vi "ACT_Loop.vi"() -> ()   [LabVIEW 2023, in "TShirtWork-SwerveDrive_ACT_ts.lvlib"]
uses:
  TShirtWork-SwerveDrive_ACT_ts.lvlib
  RoboRIO Utilities/Global_STOP.vi
  ENUM_ACT_Action.ctl
  ENUM_ACT_State.ctl
  Global_CMD_ACT_Data In.vi
  Global_ACT_Data Out.vi
  Cluster_CMD_ACT_Data.ctl
  <vilib>/Rock Robotics/WPI/MotorControl/WPI_MotorControlType.ctl
  <vilib>/Rock Robotics/SystemInterfaces/DIO/FPGA_DIOPWMChannel.ctl
  <vilib>/Rock Robotics/WPI/PWM/WPI_PWMDeadband.ctl
  <vilib>/Rock Robotics/SystemInterfaces/DIO/FPGA_DIOChannel.ctl
  <vilib>/Rock Robotics/WPI/MotorControl/WPI_MotorControlDeviceRef.ctl
  Shared Code/TypeDefs/ENUM_Module Position.ctl
  <vilib>/Rock Robotics/WPI/ThirdParty/REV Robotics/REVLib/Typedef/Spark MAX Control Type.ctl
  Type Defs/ENUM_Steer Mode Select.ctl
  Shared Code/TypeDefs/Cluster_CMD_Direction Data.ctl
  Shared Code/TypeDefs/Level_Velocity plus-minus 1.ctl
  Shared Code/TypeDefs/Dial_Compase heading unit circle CCW positive.ctl
  Shared Code/TypeDefs/Cluster_Module Velocity-Direction-Rotations.ctl
  Shared Code/TypeDefs/Cluster_Swerve 4 Steer and Velocity.ctl
  Shared Code/TypeDefs/Cluster_X-Y.ctl
  Type Defs/Cluster_Avoid Zone.ctl
  PigeonIMU/Global_SEN_Data Out.vi
  PigeonIMU/PigeonIMU_SEN_ts.lvlib
  Shared Code/TypeDefs/Cluster_Config_SwerveParam Drive.ctl
  Type Defs/Cluster_Length and Width.ctl
  Shared Code/TypeDefs/Cluster_Config_SwerveParam Steer.ctl
  Shared Code/TypeDefs/Cluster_Config_Swerve Drive Parameters.ctl
  Shared Code/TypeDefs/ENUM_CMD_Mode Select.ctl
  <vilib>/Rock Robotics/WPI/ThirdParty/Phoenix-LabVIEW/Motor Controller/Get/CTRE_Phoenix_MotorController_GetSelectedSensorData.vi
  Shared Code/TypeDefs/ENUM_Min Max Values.ctl
  Type Defs/Cluster_Zero Steer Positions.ctl
  Shared Code/TypeDefs/Dial_Actual Direction.ctl
  Shared Code/TypeDefs/Cluster_Module Actual Settings.ctl
  Shared Code/TypeDefs/Cluster_Swerve Actual Settings.ctl
panel:
  out "Yaw":T1 scale format="%.3f"
  out "Swerve SET Actual":T2 {"Back Right"."Direction" scale format="%.3f"; "Back Right"."Velocity" format="%.2f"; "Back Left"."Direction" scale format="%.3f"; "Back Left"."Velocity" format="%.2f"; "Front Left"."Direction" scale format="%.3f"; "Front Left"."Velocity" format="%.2f"; "Front Right"."Direction" scale format="%.3f"; "Front Right"."Velocity" format="%.2f"}
  out "calc time":dbl
  in  "Zero Steer Positions":T5 {"RB"."Max" format="%.3g"; "RB"."Min" format="%.3g"; "LB"."Max" format="%.3g"; "LB"."Min" format="%.3g"; "LF"."Max" format="%.3g"; "LF"."Min" format="%.3g"; "RF"."Max" format="%.3g"; "RF"."Min" format="%.3g"}
  out "Swerve Set":T7 {"Back Right"."Angle" scale format="%.3f"; "Back Right"."Velocity" scale=-1.0..1.0 scale format="%.1f"; "Back Left"."Angle" scale format="%.3f"; "Back Left"."Velocity" scale=-1.0..1.0 scale format="%.1f"; "Front Left"."Angle" scale format="%.3f"; "Front Left"."Velocity" scale=-1.0..1.0 scale format="%.1f"; "Front Right"."Angle" scale format="%.3f"; "Front Right"."Velocity" scale=-1.0..1.0 scale format="%.1f"}
  out "Max Velocity(RPM)":dbl=200.0
  out "Steer Mode":T10
  out "Max Velocity FPS":dbl=2.0
  out "Steer Position Values":dbl[](array[numeric])
  out "Drive Control Mode":T11
  in  "Stream":bool=TRUE
  out "Input CMD":T12 {"Auto Angle" scale format="%.3f"; "Direction"."Rotate(Yaw) CCW 1 CW -1" scale=1.0..-1.0; "Direction"."Traverse"."Angle" scale format="%.3f"; "Direction"."Traverse"."Velocity" scale=-1.0..1.0 scale format="%.1f"}
  out "Cycle Time (S)":dbl format="%.3g"
  # "\"Front\" of Robot"
  # "X"
  # "+CCW"
  # "Y"
  # "(0,0)"
  # "\"Front\" of Robot"
  # "Right Hand Rule"
  # "X"
  # "+CCW"
  # "Y"
  # "(0,0)"
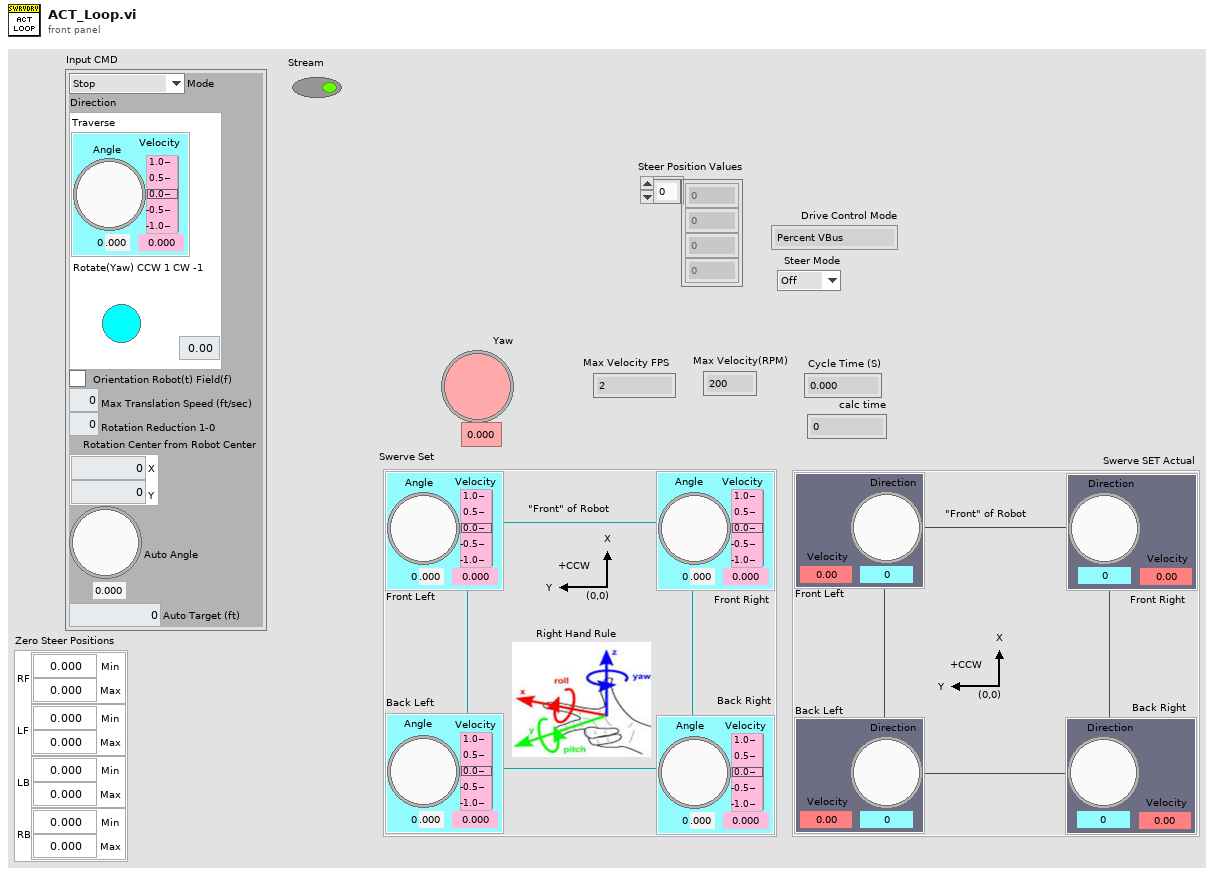
[diagram p1: front panel]
types:
  T1 = typedef "Dial_Compase heading unit circle CCW positive.ctl" = dbl
  T2 = typedef "Cluster_Swerve Actual Settings.ctl" = cluster{"Front Right":T3, "Front Left":T3, "Back Left":T3, "Back Right":T3}
  T3 = typedef "Cluster_Module Actual Settings.ctl" = cluster{"Velocity":dbl, "Direction":T4, "Encoder":dbl}
  T4 = typedef "Dial_Actual Direction.ctl" = dbl
  T5 = typedef "Cluster_Zero Steer Positions.ctl" = cluster{"RF":T6, "LF":T6, "LB":T6, "RB":T6}
  T6 = typedef "ENUM_Min Max Values.ctl" = cluster{"Min":dbl, "Max":dbl}
  T7 = typedef "Cluster_Swerve 4 Steer and Velocity.ctl" = cluster{"Front Right":T8, "Front Left":T8, "Back Left":T8, "Back Right":T8}
  T8 = typedef "Cluster_Module Velocity-Direction-Rotations.ctl" = cluster{"Velocity":T9, "Angle":T1, "Rotations Count":dbl}
  T9 = typedef "Level_Velocity plus-minus 1.ctl" = dbl
  T10 = typedef "ENUM_Steer Mode Select.ctl" = enum16{"Off", "Hold", "Steer"}
  T11 = typedef "Spark MAX Control Type.ctl" = enum16{"Percent VBus", "Voltage", "Velocity", "Position", "Smart Motion", "Current", "Smart Velocity"}
  T12 = typedef "TShirtWork-SwerveDrive_ACT_ts.lvlib/Cluster_CMD_ACT_Data.ctl" = cluster{"Mode":T13, "Direction":T14, "Orientation Robot(t) Field(f)":bool, "Max Translation Speed (ft/sec)":dbl, "Rotation Reduction 1-0":dbl, "Rotation Center from Robot Center":T15, "Auto Angle":T1, "Auto Target (ft)":dbl}
  T13 = typedef "ENUM_CMD_Mode Select.ctl" = enum16{"Stop", "Move", "Turret Manual"}
  T14 = typedef "Cluster_CMD_Direction Data.ctl" = cluster{"Traverse":T8, "Rotate(Yaw) CCW 1 CW -1":dbl}
  T15 = typedef "Cluster_X-Y.ctl" = cluster{"X":dbl, "Y":dbl}
  T16 = typedef "Cluster_Config_Swerve Drive Parameters.ctl" = cluster{"SwerveParam Ver":u64, "Frame":T17, "Steer":T18, "Drive":T19}
  T17 = typedef "Cluster_Length and Width.ctl" = cluster{"Length":dbl, "Width":dbl}
  T18 = typedef "Cluster_Config_SwerveParam Steer.ctl" = cluster{"CPR":dbl}
  T19 = typedef "Cluster_Config_SwerveParam Drive.ctl" = cluster{"CPR":dbl, "RevMotor/Wheel":dbl, "Wheel Diameter (in)":dbl}
  T20 = typedef "Cluster_Avoid Zone.ctl" = cluster{"pos 1":dbl, "pos 2":dbl}
  T21 = typedef "ENUM_Module Position.ctl" = enum16{"Left-Front", "Right-Front", "Left-Back", "Right-Back"}
  T22 = typedef "WPI_MotorControlDeviceRef.ctl" = cluster{"DeviceStatus":errorcluster, "Type":T23, "PWM":cluster{"PWM Channel":T24, "DeadBand":T25}, "CAN":cluster{"Device Number":u8, "SetOutput VI Ref":variant, "GetOutput VI Ref":variant, "Enable VI Ref":variant, "Disable VI Ref":variant, "Data":variant}, "Invert":bool, "DIO PWM":cluster{"PWM \"Enable\" Channel":T24, "DIOChannel":T26, "PWM Rate":dbl}}
  T23 = typedef "WPI_MotorControlType.ctl" = enum16{"PWM", "CAN", "DIO PWM"}
  T24 = typedef "FPGA_DIOPWMChannel.ctl" = enum8{"PWM 0", "PWM 1", "PWM 2", "PWM 3", "PWM 4", "PWM 5", "PWM 6", "PWM 7", "PWM 8", "PWM 9", "PWM MXP 0", "PWM MXP 1", "PWM MXP 2", "PWM MXP 3", "PWM MXP 4", "PWM MXP 5", "PWM MXP 6", "PWM MXP 7", "PWM MXP 8", "PWM MXP 9", "Invalid"}
  T25 = typedef "WPI_PWMDeadband.ctl" = cluster{"Name":string, "maxPositivePwm":i32, "minPositivePwm":i32, "centerPwm":i32, "maxNegativePwm":i32, "minNegativePwm":i32, "angularRange":u16}
  T26 = typedef "FPGA_DIOChannel.ctl" = enum8{"DIO 0", "DIO 1", "DIO 2", "DIO 3", "DIO 4", "DIO 5", "DIO 6", "DIO 7", "DIO 8", "DIO 9", "DIO MXP 0", "DIO MXP 1", "DIO MXP 2", "DIO MXP 3", "DIO MXP 4", "DIO MXP 5", "DIO MXP 6", "DIO MXP 7", "DIO MXP 8", "DIO MXP 9", "DIO MXP 10", "DIO MXP 11", "DIO MXP 12", "DIO MXP 13", "DIO MXP 14", "DIO MXP 15", "SPI Port CS1", "SPI Port CS2", "SPI Port CS3", "SPI Port MISO", "SPI Port MOSI", "Invalid"}
  T27 = typedef "TShirtWork-SwerveDrive_ACT_ts.lvlib/ENUM_ACT_State.ctl" = enum16{"Startup", "Stopping", "Moving", "Shutdown"}
  T28 = typedef "TShirtWork-SwerveDrive_ACT_ts.lvlib/ENUM_ACT_Action.ctl" = enum16{"No Action", "Reset Time", "Reset All", "2 Pos Set Direction", "2 Pos Set Speed", "Record Data", "Set Move from Values"}
  T29 = cluster{"Motor List":T21[], "Drive Refs":T22[], "Steer Refs":T22[], "State":T27, "Previous State":T27, "Current Time":timestamp, "Previous Time":timestamp, "Start Time":timestamp, "Target Time (ms)":u32, "Cycle Time(S)":dbl, "ACT Input":T12, "Drive Control Mode":T11, "Drive PID Slot":i32, "Steer Position Values":dbl[], "Drive Velocity Values":dbl[], "Steer Position Times":dbl[], "Drive Velocity Times":dbl[], "Stream":bool, "Drive Output Times":dbl[], "Drive Output Values":dbl[], "Zero Start Steer Positions":dbl[], "Steer Mode":T10, "Max Velocity RPM":dbl, "Avoid Zone":T20, "Swerve Set":T7, "calc Start Time":dbl, "Compass Heading":T1, "Swerve Config ":T16, "Team Folder":path}
  T30 = typedef "SwerveDrive_ACT_ts.lvlib/Cluster_CMD_ACT_Data.ctl" = cluster{"Mode":T13, "Direction":T14, "Orientation Robot(t) Field(f)":bool, "Max Translation Speed (ft/sec)":dbl, "Rotation Reduction 1-0":dbl, "Rotation Center from Robot Center":T15, "Auto Angle":T1, "Auto Target (ft)":dbl}
  T31 = typedef "Cluster_Unity Yaw-Pitch-Roll.ctl" = cluster{"Yaw":T1, "Pitch":T1, "Roll":T1}
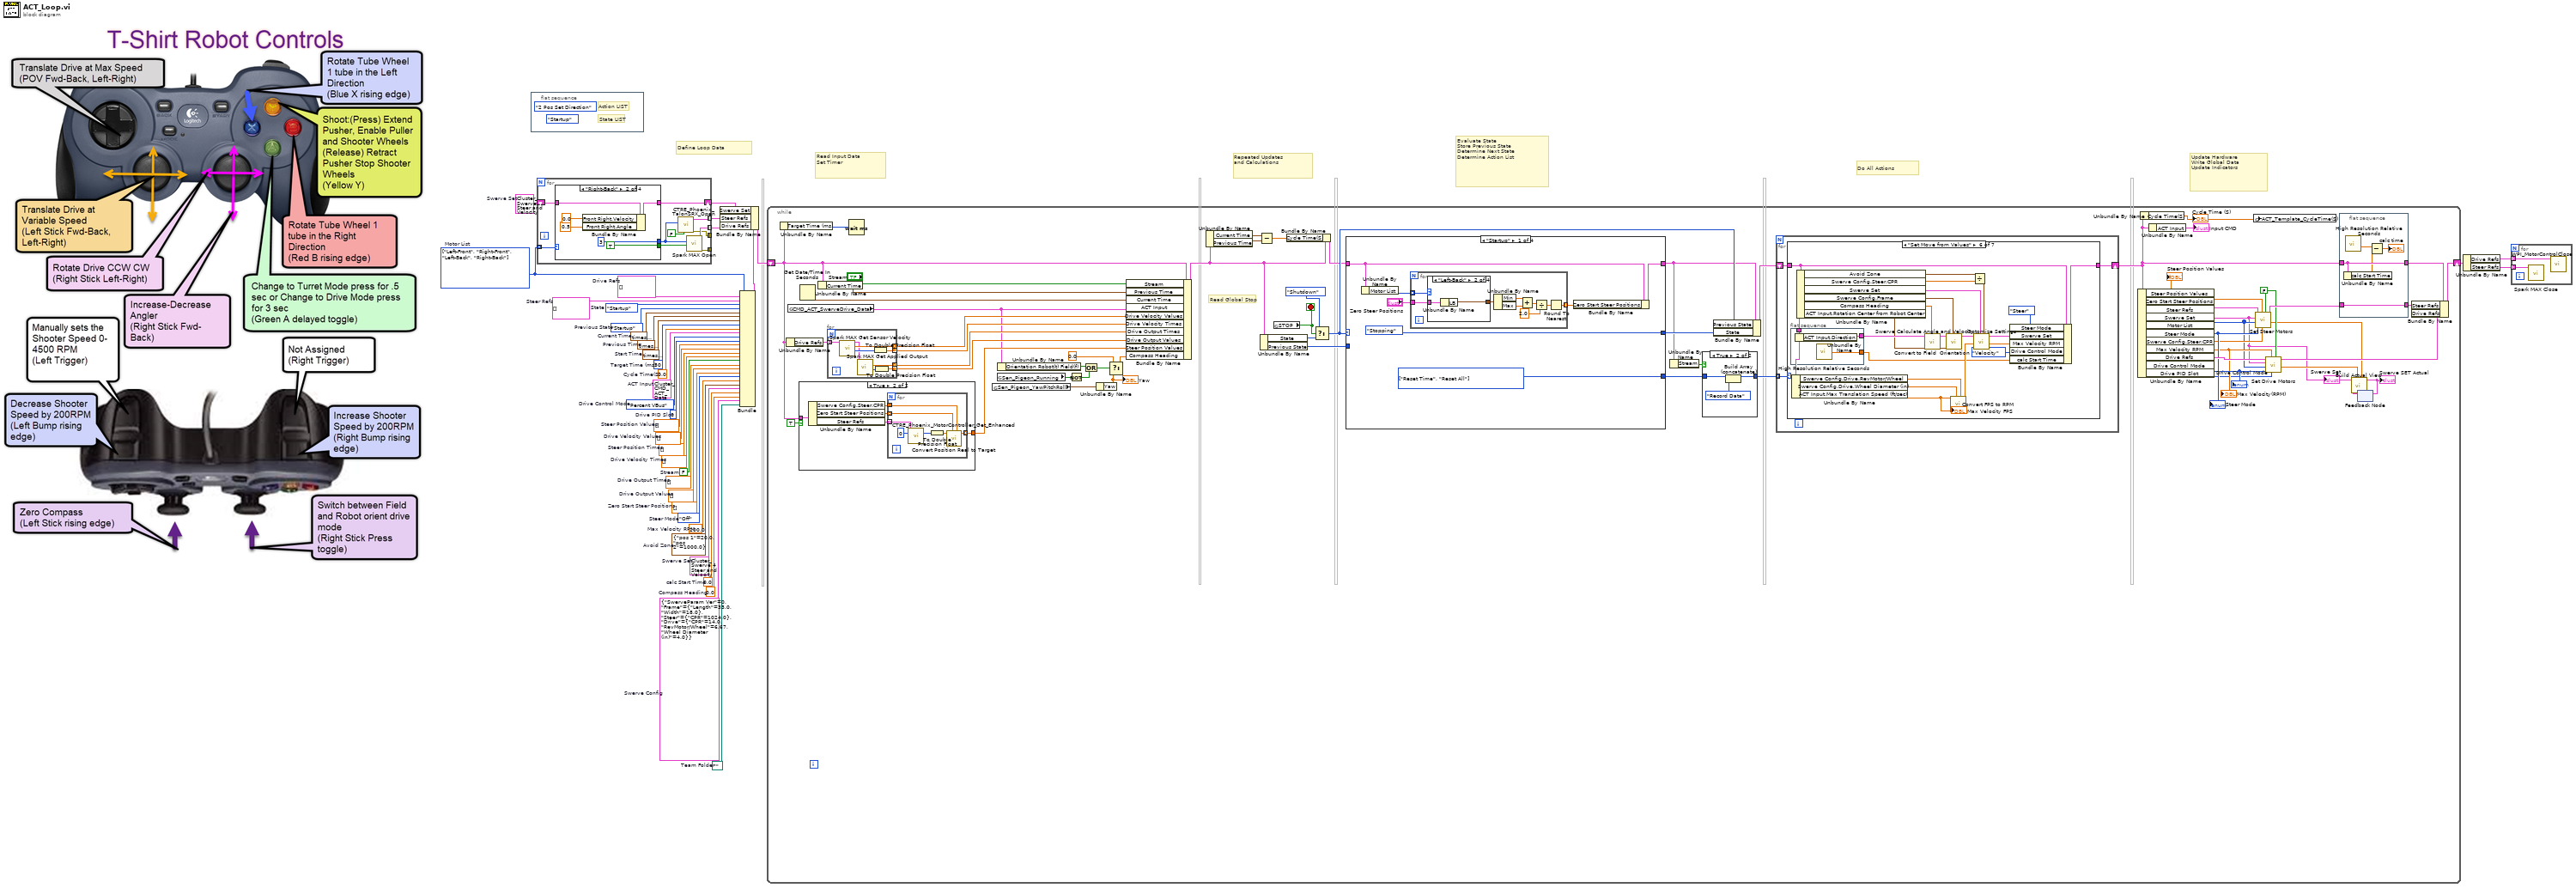
[diagram p0: block diagram]
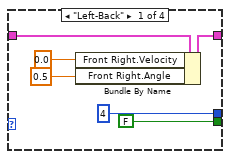
[diagram p2: hidden frame]
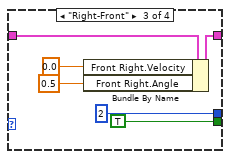
[diagram p3: hidden frame]
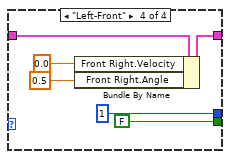
[diagram p4: hidden frame]
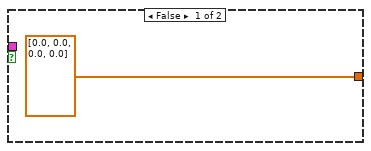
[diagram p5: hidden frame]
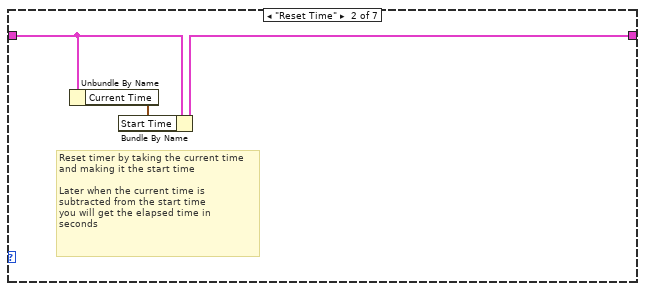
[diagram p8: hidden frame]
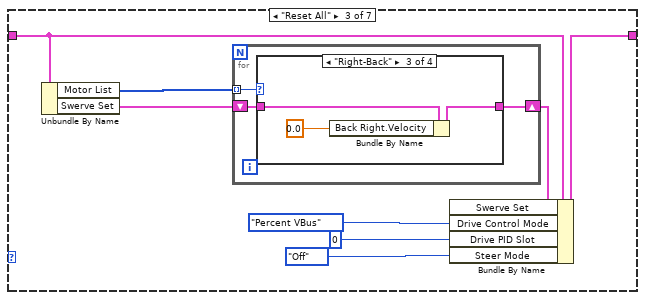
[diagram p9: hidden frame]
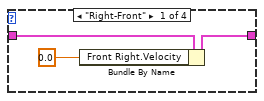
[diagram p10: hidden frame]
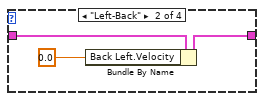
[diagram p11: hidden frame]
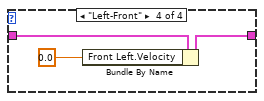
[diagram p12: hidden frame]
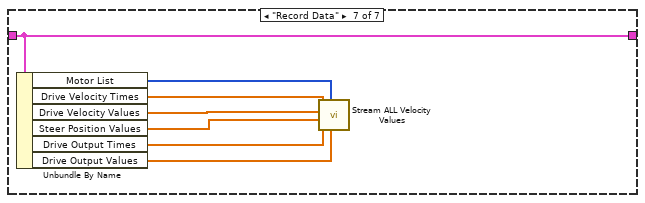
[diagram p15: hidden frame]
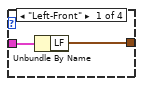
[diagram p16: hidden frame]
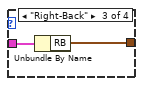
[diagram p17: hidden frame]
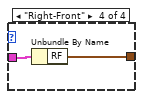
[diagram p18: hidden frame]
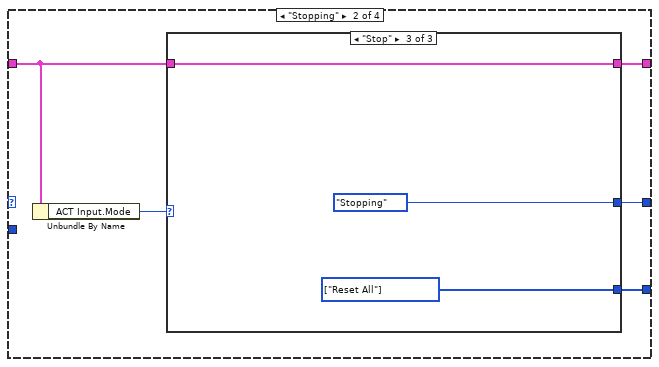
[diagram p19: hidden frame]
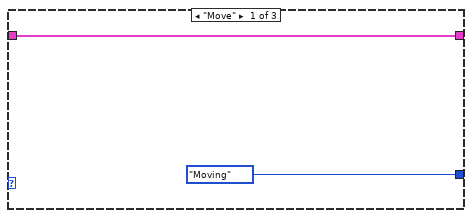
[diagram p20: hidden frame]
diagram:
  w1 = path ""  # Team Folder
  w2 = T16 {"SwerveParam Ver"=0, "Frame"={"Length"=33.0, "Width"=18.0}, "Steer"={"CPR"=1024.0}, "Drive"={"CPR"=14.0, "RevMotor/Wheel"=6.67, "Wheel Diameter (in)"=4.0}}  # Swerve Config
  w3 = T1 0.0  # Compass Heading
  w4 = 0.0  # calc Start Time
  w6 = T7 {"Front Right"={"Velocity"=0.0, "Angle"=0.0, "Rotations Count"=0.0}, "Front Left"={"Velocity"=0.0, "Angle"=0.0, "Rotations Count"=0.0}, "Back Left"={"Velocity"=0.0, "Angle"=0.0, "Rotations Count"=0.0}, "Back Right"={"Velocity"=0.0, "Angle"=0.0, "Rotations Count"=0.0}}  # Swerve Set
  w7 = T7 {"Front Right"={"Velocity"=0.0, "Angle"=0.0, "Rotations Count"=0.0}, "Front Left"={"Velocity"=0.0, "Angle"=0.0, "Rotations Count"=0.0}, "Back Left"={"Velocity"=0.0, "Angle"=0.0, "Rotations Count"=0.0}, "Back Right"={"Velocity"=0.0, "Angle"=0.0, "Rotations Count"=0.0}}  # Swerve Set
  w8 = T20 {"pos 1"=20.0, "pos 2"=1000.0}  # Avoid Zone
  w9 = T21[] [enum."Left-Front", enum."Right-Front", enum."Left-Back", enum."Right-Back"] items=["Left-Front", "Right-Front", "Left-Back", "Right-Back"]  # Motor List
  w10 = 200.0  # Max Velocity RPM
  w11 = ENUM_Steer_Mode_Select."Off"  # Steer Mode
  w12 = dbl[] []  # Zero Start Steer Positions
  w13 = dbl[] []  # Drive Output Values
  w14 = dbl[] []  # Drive Output Times
  w15 = FALSE  # Stream
  w16 = dbl[] []  # Drive Velocity Times
  w17 = dbl[] []  # Steer Position Times
  w18 = dbl[] []  # Drive Velocity Values
  w19 = dbl[] []  # Steer Position Values
  w22 = 0  # Drive PID Slot
  w23 = Spark_MAX_Control_Type."Percent VBus"  # Drive Control Mode
  w28 = T22[] []  # Drive Refs
  w29 = T22[] []  # Steer Refs
  w31 = 0.0  # Cycle Time(S)
  w32 = ENUM_ACT_State."Startup"  # Previous State
  w33 = timestamp(0 s since 1904-01-01)  # Previous Time
  w34 = u32 50  # Target Time (ms)
  w35 = T12 {"Mode"=enum."Stop", "Direction"={"Traverse"={"Velocity"=0.0, "Angle"=0.0, "Rotations Count"=0.0}, "Rotate(Yaw) CCW 1 CW -1"=0.0}, "Orientation Robot(t) Field(f)"=FALSE, "Max Translation Speed (ft/sec)"=0.0, "Rotation Reduction 1-0"=0.0, "Rotation Center from Robot Center"={"X"=0.0, "Y"=0.0}, "Auto Angle"=0.0, "Auto Target (ft)"=0.0}  # ACT Input
  w36 = timestamp(0 s since 1904-01-01)  # Start Time
  w37 = timestamp(0 s since 1904-01-01)  # Current Time
  w38 = ENUM_ACT_State."Startup"  # State
  # "Define Loop Data"
  # "Repeated Updates\nand Calculations"
  # "Read Input Data\nSet Timer"
  # "Evaluate State\nStore Previous State\nDetermine Next State\nDetermine Action List"
  # "Do All Actions"
  # "Update Hardware\nWrite Global Data\nUpdate Indicators"
  n1 = flat-sequence {
    frame #0 {
      (unwired) ENUM_ACT_State."Startup" ("State")
      (unwired) ENUM_ACT_Action."2 Pos Set Direction" ("Action")
      # "State LIST"
      # "Action LIST"
    }
  }
  n2 = for {
    tunnel: w9 -> [w44] mode=indexing
    tunnel: [w46] -> w25 mode=indexing
    tunnel: [w45] -> w24 mode=indexing
    shift-right: [w41] -> w5
    shift-left: w6 -> [w42]
    tunnel: [w40] -> _
    tunnel: [w39] -> _
    n3 = case shown="\"Right-Back\"" w44 {
      tunnel: [FALSE ("Invert") TRUE ("Invert") TRUE ("Invert") FALSE ("Invert")] -> w47
      tunnel: [u8 4 ("unsigned 8bit integer") u8 3 ("unsigned 8bit integer") u8 2 ("unsigned 8bit integer") u8 1 ("unsigned 8bit integer")] -> w43
      tunnel: w42 -> [w50 w56 w63 w68]
      tunnel: [w49 w55 w64 w67] -> w41
      frame "Left-Back" {
        n4 = Bundle By Name(cluster=w50, "Front Right.Velocity"=T9 0.0 ("Front Right.Velocity (0-1)"), "Front Right.Angle"=T1 0.5 ("Front Right.Angle(0-1)")) -> (w49:T7)
      }
      frame "Right-Back" {
        n5 = Bundle By Name(cluster=w56, "Front Right.Velocity"=T9 0.0 ("Front Right.Velocity (0-1)"), "Front Right.Angle"=T1 0.5 ("Front Right.Angle(0-1)")) -> (w55:T7)
      }
      frame "Right-Front" {
        n6 = Bundle By Name(cluster=w63, "Front Right.Velocity"=T9 0.0 ("Front Right.Velocity (0-1)"), "Front Right.Angle"=T1 0.5 ("Front Right.Angle(0-1)")) -> (w64:T7)
      }
      frame "Left-Front" {
        n7 = Bundle By Name(cluster=w68, "Front Right.Velocity"=T9 0.0 ("Front Right.Velocity (0-1)"), "Front Right.Angle"=T1 0.5 ("Front Right.Angle(0-1)")) -> (w67:T7)
      }
    }
    n8 = call <vilib>:"CTRE_Phoenix_TalonSRX_Open.vi"("Invert"=FALSE, "Device Number"=w43) -> ("error out"=w40:errorcluster, "PhoenixMotorControlDevRef"=w46:T22)  [unwired: 8 in]
    n9 = call <vilib>:"Spark MAX Open.vi"("Invert"=w47, "Device Number"=w43) -> ("error out"=w39:errorcluster, "MotorControlDeviceRef"=w45:T22)  [unwired: 8 in]
  }
  n10 = Bundle("Motor List"=w9, "Drive Refs"=w28, "Steer Refs"=w29, "State"=w38, "Previous State"=w32, "Current Time"=w37, "Previous Time"=w33, "Start Time"=w36, "Target Time (ms)"=w34, "Cycle Time(S)"=w31, "ACT Input"=w35, "Drive Control Mode"=w23, "Drive PID Slot"=w22, "Steer Position Values"=w19, "Drive Velocity Values"=w18, "Steer Position Times"=w17, "Drive Velocity Times"=w16, "Stream"=w15, "Drive Output Times"=w14, "Drive Output Values"=w13, "Zero Start Steer Positions"=w12, "Steer Mode"=w11, "Max Velocity RPM"=w10, "Avoid Zone"=w8, "Swerve Set"=w7, "calc Start Time"=w4, "Compass Heading"=w3, "Swerve Config"=w2, "Team Folder"=w1) -> (w27:T29)  [unwired: 1 in]
  n11 = Bundle By Name(cluster=w27, "Swerve Set"=w5, "Steer Refs"=w25, "Drive Refs"=w24) -> (w26:T29)
  n12 = while {
    shift-right: [w117] -> w30
    shift-left: w26 -> [w101]
    stop <- w130 stop-if-true
    w86 = FALSE
    # "Read Global Stop"
    n13 = Unbundle By Name(w101) -> ("Target Time (ms)"=w127:u32)
    n14 = Unbundle By Name(w101) -> ("Drive Refs"=w100:T22[])
    n15 = global read "Global_CMD_ACT_Data In.vi" "CMD_ACT_SwerveDrive_Data"() -> (w82:T30)
    n16 = case shown="True" TRUE {
      tunnel: [dbl[] [0.0, 0.0, 0.0, 0.0] w144] -> w102
      tunnel: w101 -> [_ w143]
      frame False {
      }
      frame True {
        n17 = Unbundle By Name(w143) -> ("Swerve Config.Steer.CPR"=w140:dbl, "Zero Start Steer Positions"=w141:dbl[], "Steer Refs"=w142:T22[])
        n18 = for {
          tunnel: w142 -> [w151] mode=indexing
          tunnel: w141 -> [w147] mode=indexing
          tunnel: [w146] -> w144 mode=indexing
          tunnel: w140 -> [w145]
          n19 = call-poly <vilib>:"CTRE_Phoenix_MotorController_Get_Enhanced.vi"("PhoenixMotorControlDevRef"=w151, "pidLoopIdx"=u32 0) -> ("Position (Raw Sensor Units)"=w149:i32)  [unwired: 10 in, 3 out]
          n20 = To Double Precision Float(number=w149) -> (double precision float=w148:dbl)
          n21 = call "Convert Position Real to Target.vi"("PPR"=w145, "Zero Value"=w147, "Real Position"=w148) -> ("Position (0-1)"=w146:dbl)  [unwired: 7 in, 1 out]
        }
      }
    }
    n22 = Get Date/Time In Seconds() -> (seconds since 1Jan1904=w133:timestamp)
    n23 = Unbundle By Name(w101) -> ("Current Time"=w126:timestamp)
    n24 = for {
      tunnel: w100 -> [w159] mode=indexing
      tunnel: [w158] -> w112 mode=indexing
      tunnel: [w156] -> w111 mode=indexing
      tunnel: [w154] -> w109 mode=indexing
      tunnel: [w152] -> w108 mode=indexing
      n25 = call <vilib>:"Spark MAX Get Sensor Velocity.vi"("MotorControlDevRef in"=w159) -> ("Timestamp"=w157:u32, "Sensor Velocity"=w158:dbl, "MotorControlDevRef out"=w155:T22)  [unwired: 7 in, 1 out]
      n26 = call <vilib>:"Spark MAX Get Applied Output.vi"("MotorControlDevRef in"=w155) -> ("Timestamp"=w153:u32, "Applied Output"=w154:dbl)  [unwired: 7 in, 2 out]
      n27 = To Double Precision Float(number=w157) -> (double precision float=w156:dbl)
      n28 = To Double Precision Float(number=w153) -> (double precision float=w152:dbl)
    }
    n29 = Wait (ms)(milliseconds to wait=w127) -> ()  [unwired: 1 out]
    n30 = global read "Global_SEN_Data Out.vi" "Sen_Pigeon_YawPitchRoll"() -> (w79:T31)
    n31 = global read "Global_SEN_Data Out.vi" "Sen_Pigeon_Running"() -> (w75:bool)
    n32 = Unbundle By Name(w82) -> ("Orientation Robot(t) Field(f)"=w81:bool)
    n33 = Not(x=w75) -> (.not. x?=w74:bool)
    n34 = Or(x=w81, y=w74) -> (x .or. y?=w76:bool)
    n35 = Unbundle By Name(w79) -> ("Yaw"=w78:T1)
    "Yaw" <- w78
    n36 = Select(t=T1 0.0, s=w76, f=w78) -> (s? t:f=w80:T1)
    n37 = Bundle By Name(cluster=w101, "Stream"="Stream", "Previous Time"=w126, "Current Time"=w133, "ACT Input"=w82, "Drive Velocity Values"=w112, "Drive Velocity Times"=w111, "Drive Output Times"=w109, "Drive Output Values"=w108, "Steer Position Values"=w102, "Compass Heading"=w80) -> (w121:T29)
    n38 = Unbundle By Name(w121) -> ("Current Time"=w122:timestamp, "Previous Time"=w123:timestamp)
    n39 = Subtract(x=w122, y=w123) -> (x-y=w119:dbl)
    n40 = Unbundle By Name(w121) -> ("State"=w128:T27, "Previous State"=w125:T27)
    n41 = global read "Global_STOP.vi" "STOP"() -> (w130:bool)
    n42 = Bundle By Name(cluster=w121, "Cycle Time(S)"=w119) -> (w120:T29)
    n43 = Select(t=ENUM_ACT_State."Shutdown" ("State"), s=w130, f=w128) -> (s? t:f=w124:T27)
    n44 = case shown="\"Startup\"" w124 {
      tunnel: w120 -> [w229 w252 w264 w280]
      tunnel: [w230 w253 w265 w280] -> w107
      tunnel: [ENUM_ACT_State."Stopping" ("State") w254 w266 ENUM_ACT_State."Shutdown" ("State")] -> w131
      tunnel: [w232 w250 w262 w278] -> w105
      tunnel: w125 -> [_ _ _ _]
      frame "Startup" {
        w232 = T28[] [enum."Reset Time", enum."Reset All"] items=["No Action", "Reset Time", "Reset All", "2 Pos Set Direction", "2 Pos Set Speed", "Record Data", "Set Move from Values"] ("Actions")
        n45 = Unbundle By Name(w229) -> ("Motor List"=w228:T21[])
        n46 = for {
          tunnel: w228 -> [w241] mode=indexing
          tunnel: "Zero Steer Positions" -> [w240]
          tunnel: [w233] -> w226 mode=indexing
          n47 = case shown="\"Left-Back\"" w241 {
            tunnel: w240 -> [w243 w245 w247 w249]
            tunnel: [w242 w244 w246 w248] -> w239
            frame "Left-Front" {
              n48 = Unbundle By Name(w243) -> ("LF"=w242:T6)
            }
            frame "Left-Back" {
              n49 = Unbundle By Name(w245) -> ("LB"=w244:T6)
            }
            frame "Right-Back" {
              n50 = Unbundle By Name(w247) -> ("RB"=w246:T6)
            }
            frame "Right-Front" {
              n51 = Unbundle By Name(w249) -> ("RF"=w248:T6)
            }
          }
          n52 = Unbundle By Name(w239) -> ("Min"=w237:dbl, "Max"=w238:dbl)
          n53 = Add(x=w237, y=w238) -> (x+y=w236:dbl)
          n54 = Divide(x=w236, y=2.0) -> (x/y=w234:dbl)
          n55 = Round To Nearest(number=w234) -> (nearest integer value=w233:dbl)
        }
        n56 = Bundle By Name(cluster=w229, "Zero Start Steer Positions"=w226) -> (w230:T29)
      }
      frame "Stopping" {
        n57 = Unbundle By Name(w252) -> ("ACT Input.Mode"=w251:T13)
        n58 = case shown="\"Stop\"" w251 {
          tunnel: [ENUM_ACT_State."Moving" ("State") ENUM_ACT_State."Moving" ("State") ENUM_ACT_State."Stopping" ("State")] -> w254
          tunnel: [w255 w257 w260] -> w253
          tunnel: w252 -> [w255 w257 w260]
          tunnel: [_ _ w259] -> w250
          frame "Move" {
          }
          frame "Turret Manual" {
          }
          frame "Stop" {
            w259 = T28[] [enum."Reset All"] items=["No Action", "Reset Time", "Reset All", "2 Pos Set Direction", "2 Pos Set Speed", "Record Data", "Set Move from Values"] ("Actions")
          }
        }
      }
      frame "Moving" {
        n59 = Unbundle By Name(w264) -> ("ACT Input.Mode"=w263:T13)
        n60 = case shown="\"Turret Manual\"" w263 {
          tunnel: [ENUM_ACT_State."Moving" ("State") ENUM_ACT_State."Moving" ("State") ENUM_ACT_State."Stopping" ("State")] -> w266
          tunnel: [w268 w271 w276] -> w265
          tunnel: w264 -> [w268 w270 w276]
          tunnel: [w267 w273 w275] -> w262
          frame "Move" {
            w267 = T28[] [enum."Set Move from Values"] items=["No Action", "Reset Time", "Reset All", "2 Pos Set Direction", "2 Pos Set Speed", "Record Data", "Set Move from Values"] ("Actions")
          }
          frame "Turret Manual" {
            w273 = T28[] [enum."Set Move from Values"] items=["No Action", "Reset Time", "Reset All", "2 Pos Set Direction", "2 Pos Set Speed", "Record Data", "Set Move from Values"] ("Actions")
            n61 = Bundle By Name(cluster=w270, "ACT Input.Direction.Traverse.Velocity"=T9 0.0) -> (w271:T29)
          }
          frame "Stop" {
            w275 = T28[] [enum."Reset All"] items=["No Action", "Reset Time", "Reset All", "2 Pos Set Direction", "2 Pos Set Speed", "Record Data", "Set Move from Values"] ("Actions")
          }
        }
      }
      frame "Shutdown" {
        w278 = T28[] [enum."Reset All"] items=["No Action", "Reset Time", "Reset All", "2 Pos Set Direction", "2 Pos Set Speed", "Record Data", "Set Move from Values"] ("Actions")
      }
    }
    n62 = Unbundle By Name(w107) -> ("Stream"=w106:bool)
    n63 = case shown="True" w106 {
      tunnel: w105 -> [w160 w163]
      tunnel: [w160 w162] -> w104
      frame False {
      }
      frame True {
        n64 = Build Array (concatenate)(w163, ENUM_ACT_Action."Record Data" ("Action")) -> (w162:T28[])
      }
    }
    n65 = Bundle By Name(cluster=w107, "Previous State"=w124, "State"=w131) -> (w132:T29)
    n66 = for {
      tunnel: w104 -> [w166] mode=indexing
      shift-right: [w165] -> w89
      shift-left: w132 -> [w164]
      n67 = case shown="\"Set Move from Values\"" w166 {
        tunnel: w164 -> [w167 w170 w175 w194 w195 w211 w225]
        tunnel: [w167 w169 w178 w194 w195 w215 w225] -> w165
        frame "No Action" {
        }
        frame "Reset Time" {
          # "Reset timer by taking the current time\nand making it the start time\n\nLater when the current time is \nsubtracted from the start time\nyou will get the elapsed time in \nseconds"
          n68 = Unbundle By Name(w170) -> ("Current Time"=w168:timestamp)
          n69 = Bundle By Name(cluster=w170, "Start Time"=w168) -> (w169:T29)
        }
        frame "Reset All" {
          n70 = Unbundle By Name(w175) -> ("Motor List"=w173:T21[], "Swerve Set"=w172:T7)
          n71 = for {
            tunnel: w173 -> [w181] mode=indexing
            shift-right: [w179] -> w171
            shift-left: w172 -> [w180]
            n72 = case shown="\"Right-Back\"" w181 {
              tunnel: w180 -> [w184 w187 w190 w193]
              tunnel: [w183 w186 w189 w192] -> w179
              frame "Right-Front" {
                n73 = Bundle By Name(cluster=w184, "Front Right.Velocity"=T9 0.0 ("Front Right.Velocity (0-1)")) -> (w183:T7)
              }
              frame "Left-Back" {
                n74 = Bundle By Name(cluster=w187, "Back Left.Velocity"=T9 0.0 ("Front Right.Velocity (0-1)")) -> (w186:T7)
              }
              frame "Right-Back" {
                n75 = Bundle By Name(cluster=w190, "Back Right.Velocity"=T9 0.0 ("Front Right.Velocity (0-1)")) -> (w189:T7)
              }
              frame "Left-Front" {
                n76 = Bundle By Name(cluster=w193, "Front Left.Velocity"=T9 0.0 ("Front Right.Velocity (0-1)")) -> (w192:T7)
              }
            }
          }
          n77 = Bundle By Name(cluster=w175, "Swerve Set"=w171, "Drive Control Mode"=Spark_MAX_Control_Type."Percent VBus", "Drive PID Slot"=0, "Steer Mode"=ENUM_Steer_Mode_Select."Off") -> (w178:T29)
        }
        frame "2 Pos Set Direction" {
        }
        frame "2 Pos Set Speed" {
        }
        frame "Set Move from Values" {
          n78 = flat-sequence {
            tunnel: w211 -> [w218]
            tunnel: [w217] -> w199
            tunnel: [w216] -> w201
            frame #0 {
              n79 = Unbundle By Name(w218) -> ("ACT Input.Direction"=w217:T14)
              n80 = call <vilib>:"High Resolution Relative Seconds.vi"() -> ("relative seconds"=w216:dbl)
            }
          }
          n81 = Unbundle By Name(w211) -> ("Swerve Config.Drive.RevMotor/Wheel"=w209:dbl, "Swerve Config.Drive.Wheel Diameter (in)"=w210:dbl, "ACT Input.Max Translation Speed (ft/sec)"=w197:dbl)
          "Max Velocity FPS" <- w197
          n82 = Unbundle By Name(w211) -> ("Avoid Zone"=w207:T20, "Swerve Config.Steer.CPR"=w208:dbl, "Swerve Set"=w204:T7, "Swerve Config.Frame"=w202:T17, "Compass Heading"=w198:T1, "ACT Input.Rotation Center from Robot Center"=w196:T15)
          n83 = call "Convert to Field  Orientation.vi"("Compass Heading"=w198, "Direction in"=w199) -> ("Corrected Direction out"=w200:T14)  [unwired: 9 in]
          n84 = call "Swerve Calculate Angle and Velocity.vi"("Frame"=w202, "Rotation Center From Robot Center"=w196, "Comand Data"=w200) -> ("Swerve Request Out"=w206:T7)  [unwired: 8 in]
          n85 = call "Convert FPS to RPM.vi"("RevMotor/RevWheel"=w209, "Wheel Diameter (in)"=w210, "Translation Speed (ft/s)"=w197) -> ("Motor Speed (RPM) Out"=w212:dbl)  [unwired: 8 in]
          n86 = Divide(x=w207, y=w208) -> (x/y=w205:T20)
          n87 = call "Optomize Settings.vi"("Aviod Zone"=w205, "Previous Swerve Setting"=w204, "Swerve Request"=w206) -> ("Swerve Setting Out"=w203:T7)  [unwired: 8 in]
          n88 = Bundle By Name(cluster=w211, "Steer Mode"=ENUM_Steer_Mode_Select."Steer", "Swerve Set"=w203, "Max Velocity RPM"=w212, "Drive Control Mode"=Spark_MAX_Control_Type."Velocity", "calc Start Time"=w201) -> (w215:T29)
        }
        frame "Record Data" {
          n89 = Unbundle By Name(w225) -> ("Motor List"=w224:T21[], "Drive Velocity Times"=w223:dbl[], "Drive Velocity Values"=w222:dbl[], "Steer Position Values"=w221:dbl[], "Drive Output Times"=w220:dbl[], "Drive Output Values"=w219:dbl[])
          n90 = call "Stream ALL Velocity Values.vi"("Output Values"=w219, "Motor List"=w224, "Output Times"=w220, "Drive Target Values"=w221, "Drive Velocity Values"=w222, "Drive Times"=w223) -> ()  [unwired: 6 in]
        }
      }
    }
    n91 = Unbundle By Name(w89) -> ("Steer Position Values"=→"Steer Position Values":dbl[], "Zero Start Steer Positions"=w103:dbl[], "Steer Refs"=w115:T22[], "Swerve Set"=w73:T7, "Motor List"=w93:T21[], "Steer Mode"=w97:T10, "Swerve Config.Steer.CPR"=w94:dbl, "Max Velocity RPM"=w95:dbl, "Drive Refs"=w114:T22[], "Drive Control Mode"=w96:T11, "Drive PID Slot"=w92:i32)
    "Drive Control Mode" <- w96
    "Steer Mode" <- w97
    "Max Velocity(RPM)" <- w95
    "Swerve Set" <- w73
    n92 = Unbundle By Name(w89) -> ("Cycle Time(S)"=w116:dbl)
    "Cycle Time (S)" <- w116
    n93 = Unbundle By Name(w89) -> ("ACT Input"=→"Input CMD":T12)
    n94 = global write "Global_ACT_Data Out.vi" "ACT_Template_CycleTime(S)"(w116) -> ()
    n95 = call "Set Steer Motors.vi"("Disable"=w86, "PPR"=w94, "Offset Encoder Positions"=w103, "Steer Control Mode"=w97, "Motor List"=w93, "Swerve Data"=w73, "Steer Refs"=w115) -> ("Encoder Counts Out"=w84:dbl[], "Array Out"=w91:T22[])  [unwired: 3 in]
    n96 = call "Set Drive Motors.vi"("Disable"=w86, "Drive PID Slot"=w92, "Max Velocity(RPM)"=w95, "Drive Control Mode"=w96, "Motor List"=w93, "Swerve Data"=w73, "Drive Refs"=w114) -> ("Speeds"=w83:dbl[], "Array Out"=w113:T22[])  [unwired: 3 in]
    n97 = flat-sequence {
      tunnel: w91 -> [w138]
      tunnel: [w138] -> w90
      tunnel: w89 -> [w137]
      tunnel: [w137] -> w88
      frame #0 {
        n98 = Unbundle By Name(w137) -> ("calc Start Time"=w135:dbl)
        n99 = call <vilib>:"High Resolution Relative Seconds.vi"() -> ("relative seconds"=w136:dbl)
        n100 = Subtract(x=w136, y=w135) -> (x-y=→"calc time":dbl)
      }
    }
    n101 = feedback #1() -> (w85:T2)  [unwired: 1 in]
    n102 = call "Build Actual View.vi"("Encoder Counts Out"=w84, "Speeds"=w83, "Previous Actual"=w85, "Swerve Set"=w73) -> ("Swerve Data out"=w87:T2)  [unwired: 7 in]
    "Swerve SET Actual" <- w87
    n103 = feedback-in #1(w87) -> ()
    n104 = Bundle By Name(cluster=w88, "Steer Refs"=w90, "Drive Refs"=w113) -> (w117:T29)
  }
  n105 = Unbundle By Name(w30) -> ("Drive Refs"=w20:T22[], "Steer Refs"=w21:T22[])
  n106 = for {
    tunnel: w21 -> [w282] mode=indexing
    tunnel: w20 -> [w281] mode=indexing
    n107 = call <vilib>:"Spark MAX Close.vi"("MotorControlDeviceRef"=w282) -> ()  [unwired: 10 in, 1 out]
    n108 = call <vilib>:"WPI_MotorControlClose.vi"("MotorControlDevRef"=w281) -> ()  [unwired: 10 in, 1 out]
  }
